vi "To XML.vi"(8 "error in (no error)":errorcluster, 9 "Parent":refnum<k20>, 10 "Document":refnum<k20>, 11 "Class in":refnum<class "Class.lvclass">) -> (0 "error out":errorcluster)   [LabVIEW 2017, in "Cobertura.lvlib" / "Class.lvclass"]
uses:
  Class.lvclass
  Class.lvclass/Class.ctl
  <resource>/objmgr/DOMUserDefRef.rc
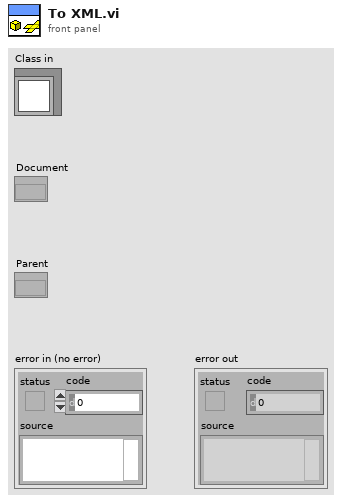
[diagram p1: front panel]
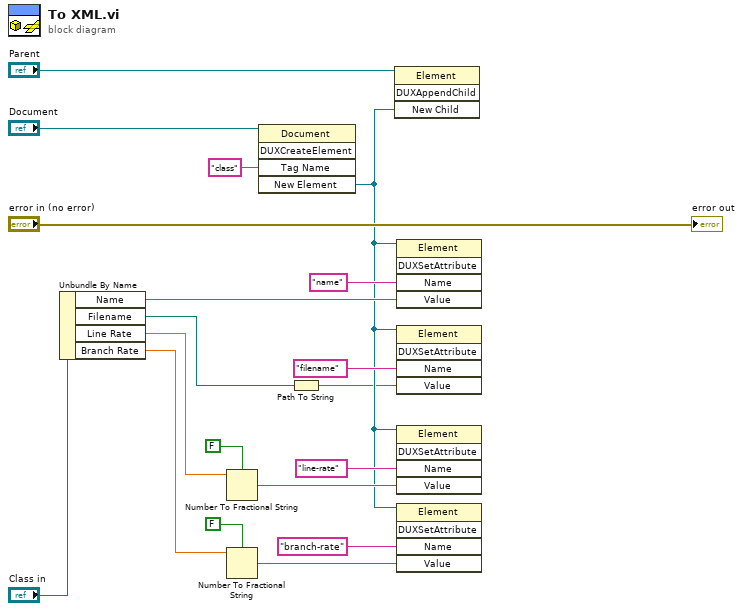
[diagram p0: block diagram]
diagram:
  n1 = Unbundle By Name("Class in") -> ("Name"=w7:string, "Filename"=w2:path, "Line Rate"=w6:dbl, "Branch Rate"=w5:dbl)
  n2 = Number To Fractional String(use system decimal point (T)=FALSE, number=w6) -> (F-format string=w16:string)  [unwired: 2 in]
  n3 = Number To Fractional String(use system decimal point (T)=FALSE, number=w5) -> (F-format string=w12:string)  [unwired: 2 in]
  n4 = invoke class="Document" method="DUXCreateElement"(reference="Document", "Tag Name"="class") -> ("New Element"=w3:refnum<k20>)  [unwired: 3 in, 4 out]
  n5 = Path To String(path=w2) -> (string=w1:string)
  n6 = invoke class="Element" method="DUXAppendChild"(reference="Parent", "New Child"=w3) -> ()  [unwired: 2 in, 4 out]
  n7 = invoke class="Element" method="DUXSetAttribute"(reference=w3, "Name"="name", "Value"=w7) -> ()  [unwired: 2 in, 5 out]
  n8 = invoke class="Element" method="DUXSetAttribute"(reference=w3, "Name"="filename", "Value"=w1) -> ()  [unwired: 2 in, 5 out]
  n9 = invoke class="Element" method="DUXSetAttribute"(reference=w3, "Name"="line-rate", "Value"=w16) -> ()  [unwired: 2 in, 5 out]
  n10 = invoke class="Element" method="DUXSetAttribute"(reference=w3, "Name"="branch-rate", "Value"=w12) -> ()  [unwired: 2 in, 5 out]
  "error out" <- "error in (no error)"
